vi "TX_ProdCons.vi"(8 "error in":errorcluster, 10 "queue in":refnum<queue>, 11 "Event Registration Refnum":refnum<event-registration>) -> (0 "error out":errorcluster)   [LabVIEW 2023]
uses:
  <vilib>/userDefined/High Color/IMAQdx.ctl
  TX_Control 3.ctl
  <vilib>/vision/Image Controls.llb/IMAQ Image.ctl
  TX_Cluster1TypeDef.ctl
  TX_EnumTypeDef.ctl
panel:
  in  "error in (no error)":errorcluster
  in  "Select Camera:":T1
  in  "EXIT":bool
  in  "Enable TCP":bool
  in  "Photo":bool
  in  "StartCam":bool
  in  "START":bool
  out "CamView":T2(plugin-control)
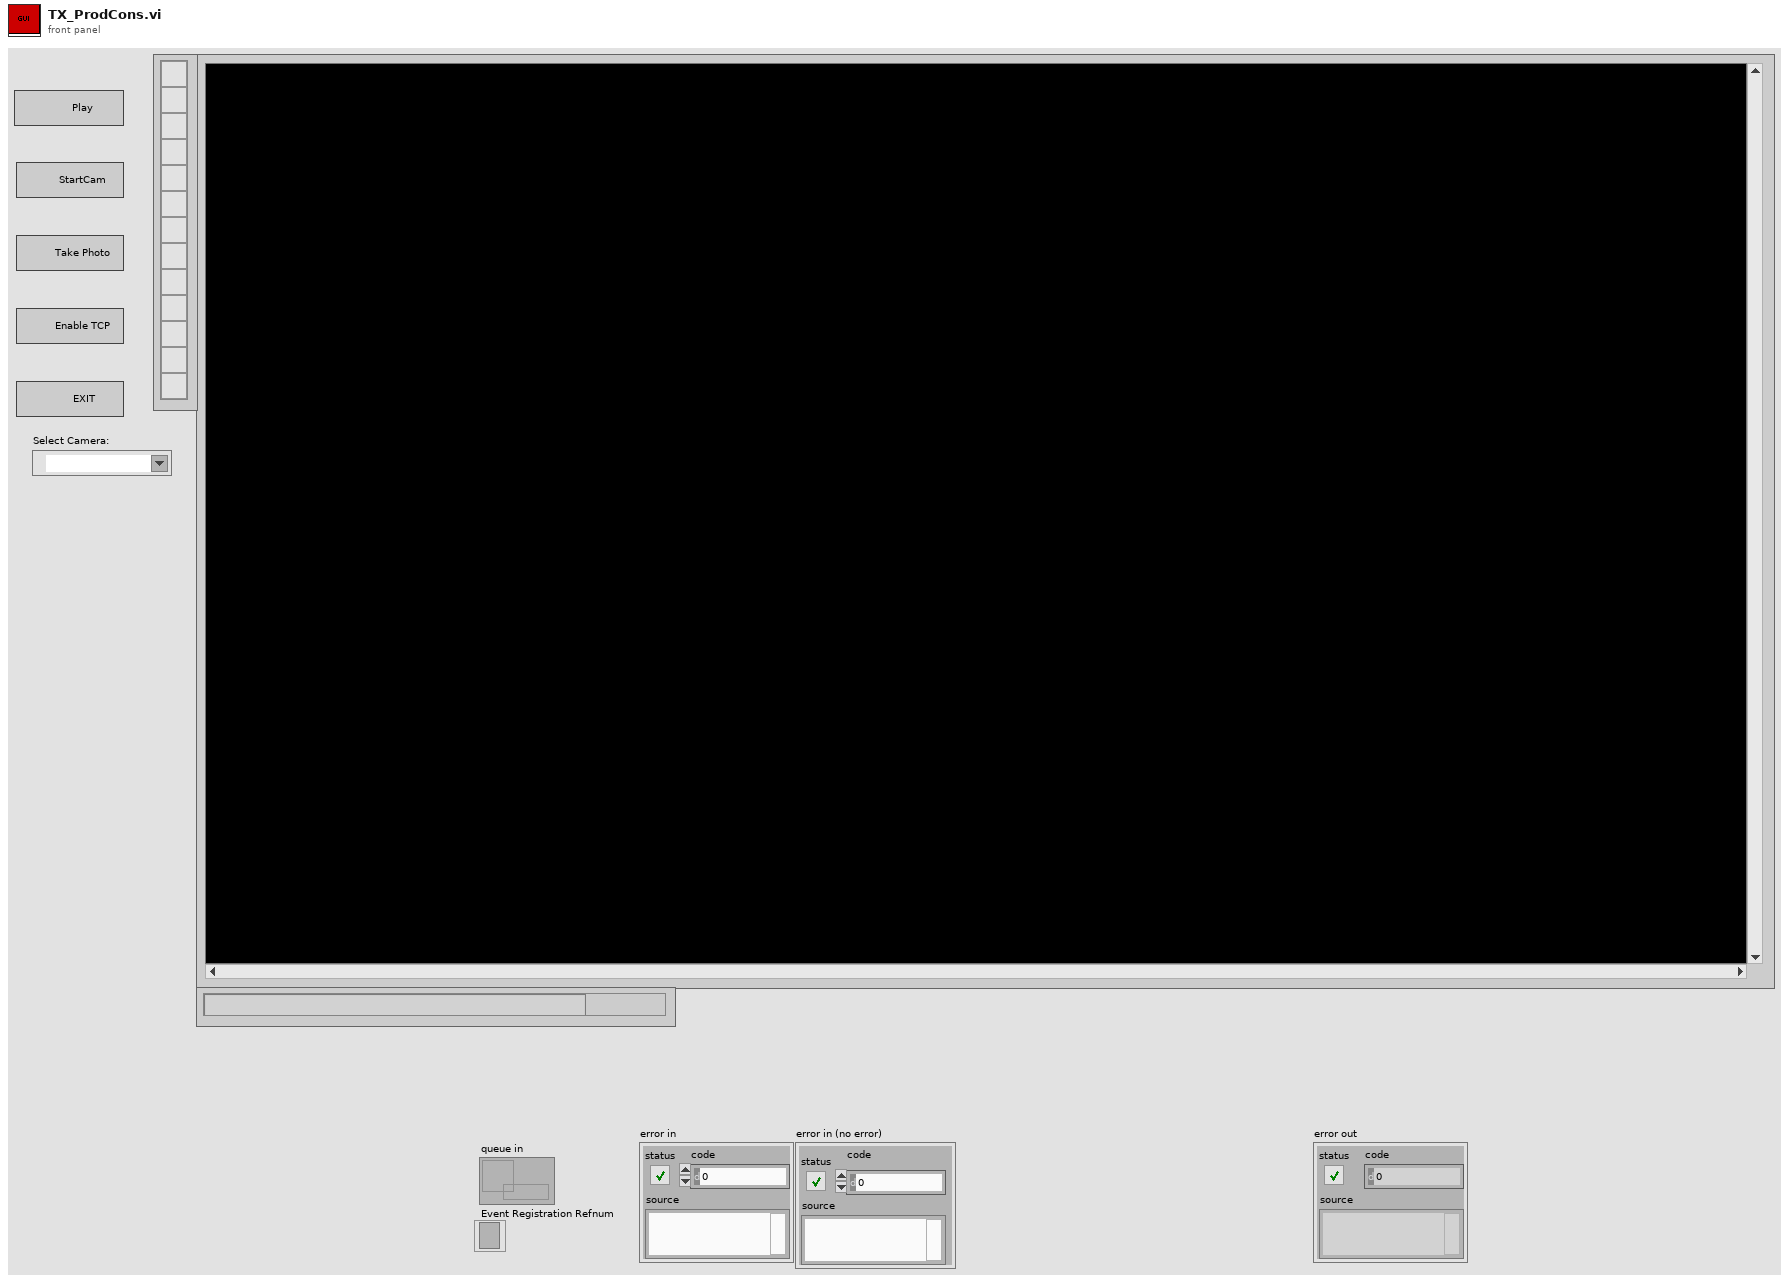
[diagram p1: front panel]
types:
  T1 = typedef "IMAQdx.ctl" = refnum<k21>
  T2 = typedef "IMAQ Image.ctl" = refnum<image>
  T3 = typedef "TX_EnumTypeDef.ctl" = enum16{"Initialize", "StartCam", "EnableTCP", "TakePhoto", "ShutDown"}
  T4 = cluster{"Enum":T3, "RawImage":T2, "Data":variant}
  T5 = typedef "TX_Cluster1TypeDef.ctl" = cluster{"Enum":T6, "CamSel":variant, "CamView":variant}
  T6 = typedef "TX_Control 3.ctl" = enum16{"Default", "StartCamera", "TakePhoto", "EnableTCP", "Cam2Display", "CloseAll"}
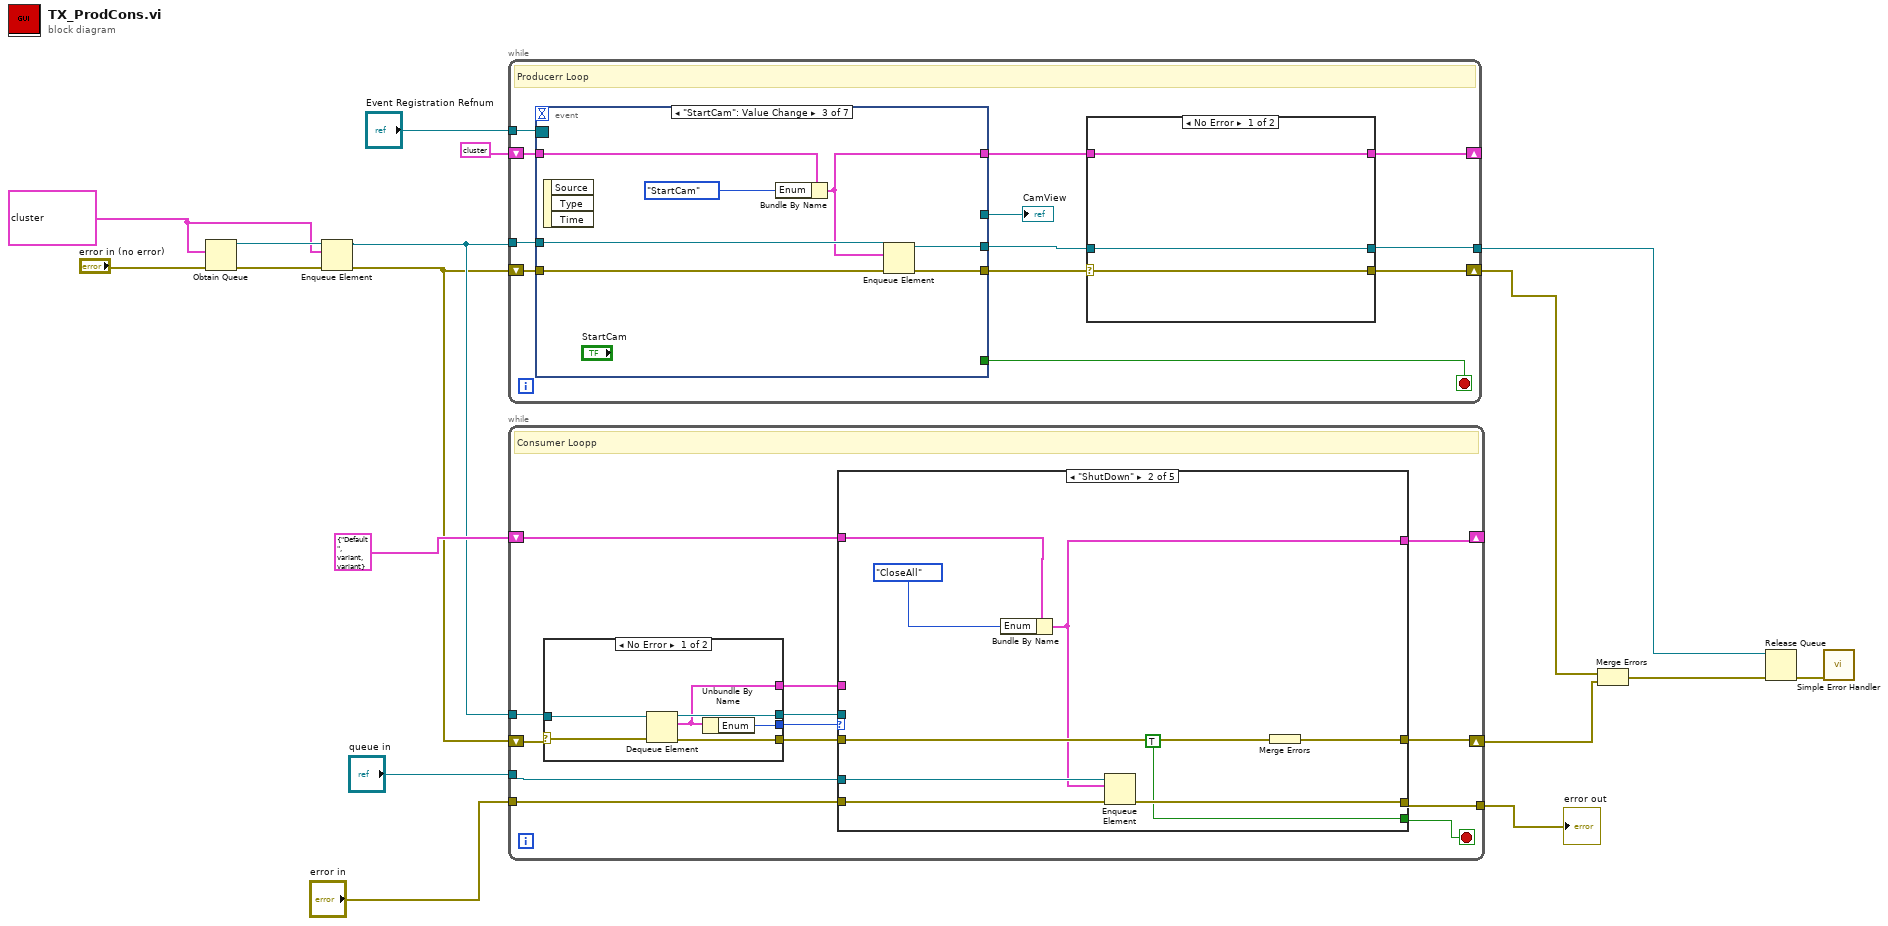
[diagram p0: block diagram]
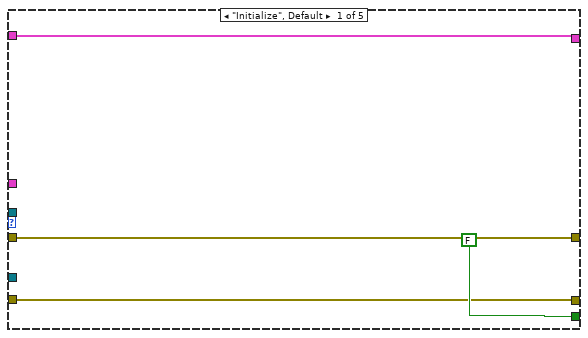
[diagram p2: hidden frame]
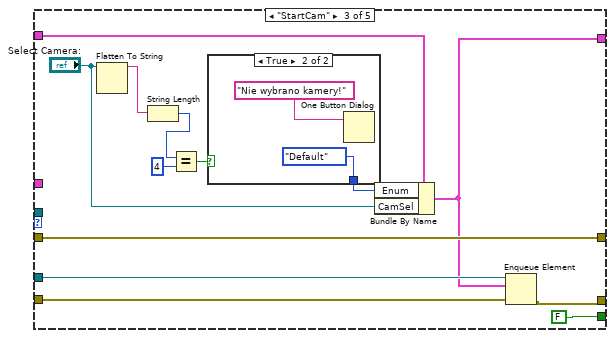
[diagram p3: hidden frame]
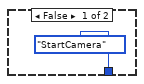
[diagram p4: hidden frame]
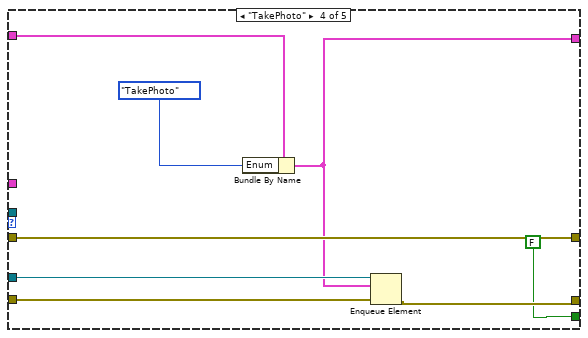
[diagram p5: hidden frame]
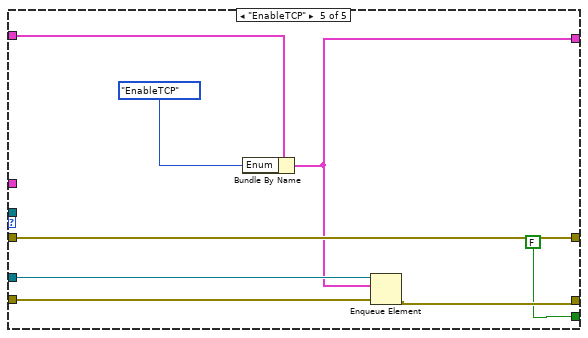
[diagram p6: hidden frame]
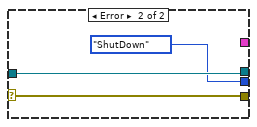
[diagram p7: hidden frame]
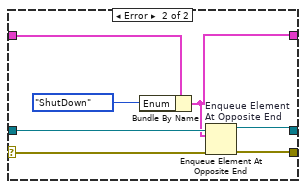
[diagram p8: hidden frame]
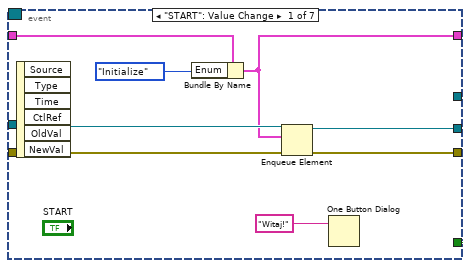
[diagram p9: hidden frame]
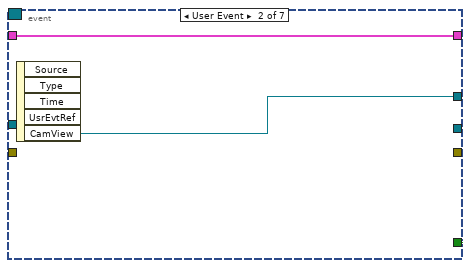
[diagram p10: hidden frame]
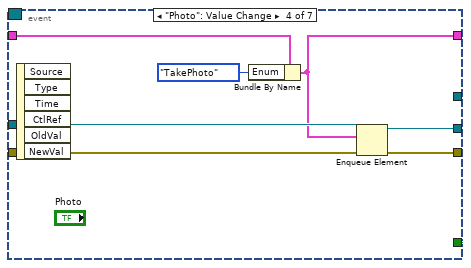
[diagram p11: hidden frame]
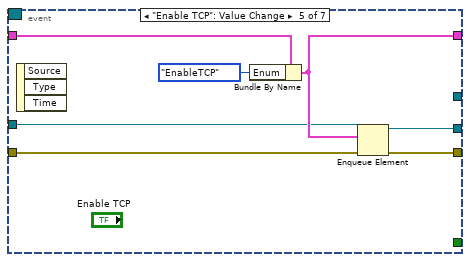
[diagram p12: hidden frame]
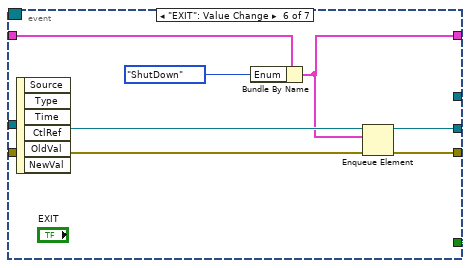
[diagram p13: hidden frame]
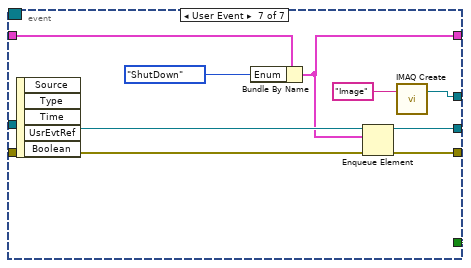
[diagram p14: hidden frame]
diagram:
  w10 = T4 {"Enum"=enum."Initialize", "RawImage"=refnum, "Data"=variant(refnum<image> refnum)} ("clusterSimple")
  n1 = Obtain Queue(element data type=w10, error in (no error)="error in (no error)") -> (queue out=w12:refnum<queue>, error out=w13:errorcluster)  [unwired: 3 in, 1 out]
  n2 = Enqueue Element(queue=w12, element=w10, error in (no error)=w13) -> (queue out=w9:refnum<queue>, error out=w8:errorcluster)  [unwired: 1 in, 1 out]
  n3 = while {
    shift-right: [w23] -> w5
    shift-left: w8 -> [w28]
    tunnel: w9 -> [w26]
    tunnel: [w24] -> w4
    tunnel: "Event Registration Refnum" -> [w22]
    shift-right: [w19] -> _
    shift-left: T4 {"Enum"=enum."Initialize", "RawImage"=refnum, "Data"=variant(refnum<image> refnum)} ("clusterSimple") -> [w21]
    stop <- w29 stop-if-true
    # "Producerr Loop"
    n4 = event shown="[2] \"StartCam\": Value Change" {
      selector: w22 -> [_ _ _ _ _ _ _]
      dyn-events: _ -> [_ _ _ _ _ _ _]
      timeout: _ -> [_ _ _ _ _ _ _]
      tunnel: [FALSE ("STOP") FALSE ("STOP") FALSE ("STOP") FALSE ("STOP") _ TRUE ("STOP") TRUE ("STOP")] -> w29
      tunnel: w28 -> [w47 _ w58 w66 w70 w82 w92]
      tunnel: [w46 _ w56 w64 w69 w81 w91] -> w27
      tunnel: w26 -> [w45 _ w59 w67 w71 w80 w90]
      tunnel: [w44 _ w57 w65 w68 w79 w89] -> w25
      tunnel: w21 -> [w43 w51 w55 w63 w72 w77 w87]
      tunnel: [w41 w51 w53 w62 w73 w75 w85] -> w20
      tunnel: [_ w49 _ _ _ _ w83] -> w18
      event "START": Value Change {
        n5 = event-data() -> ()  [unwired: 1 in, 6 out]
        n6 = Bundle By Name(cluster=w43, "Enum"=TX_EnumTypeDef."Initialize") -> (w41:T4)
        n7 = Enqueue Element(queue=w45, element=w41, error in (no error)=w47) -> (queue out=w44:refnum<queue>, error out=w46:errorcluster)  [unwired: 1 in, 1 out]
        n8 = One Button Dialog(message="Witaj!") -> ()  [unwired: 1 in, 1 out]
      }
      event User Event {
        n9 = event-data() -> ("CamView"=w49:T2)  [unwired: 1 in, 4 out]
      }
      event "StartCam": Value Change {
        n10 = event-data() -> ()  [unwired: 1 in, 3 out]
        n11 = Bundle By Name(cluster=w55, "Enum"=TX_EnumTypeDef."StartCam" ("element")) -> (w53:T4)
        n12 = Enqueue Element(queue=w59, element=w53, error in (no error)=w58) -> (queue out=w57:refnum<queue>, error out=w56:errorcluster)  [unwired: 1 in, 1 out]
      }
      event "Photo": Value Change {
        n13 = event-data() -> ()  [unwired: 1 in, 6 out]
        n14 = Bundle By Name(cluster=w63, "Enum"=TX_EnumTypeDef."TakePhoto") -> (w62:T4)
        n15 = Enqueue Element(queue=w67, element=w62, error in (no error)=w66) -> (queue out=w65:refnum<queue>, error out=w64:errorcluster)  [unwired: 1 in, 1 out]
      }
      event "Enable TCP": Value Change {
        n16 = event-data() -> ()  [unwired: 1 in, 3 out]
        n17 = Bundle By Name(cluster=w72, "Enum"=TX_EnumTypeDef."EnableTCP") -> (w73:T4)
        n18 = Enqueue Element(queue=w71, element=w73, error in (no error)=w70) -> (queue out=w68:refnum<queue>, error out=w69:errorcluster)  [unwired: 1 in, 1 out]
      }
      event "EXIT": Value Change {
        n19 = event-data() -> ()  [unwired: 1 in, 6 out]
        n20 = Bundle By Name(cluster=w77, "Enum"=TX_EnumTypeDef."ShutDown") -> (w75:T4)
        n21 = Enqueue Element(queue=w80, element=w75, error in (no error)=w82) -> (queue out=w79:refnum<queue>, error out=w81:errorcluster)  [unwired: 1 in, 1 out]
      }
      event User Event {
        n22 = event-data() -> ()  [unwired: 1 in, 5 out]
        n23 = Bundle By Name(cluster=w87, "Enum"=TX_EnumTypeDef."ShutDown") -> (w85:T4)
        n24 = Enqueue Element(queue=w90, element=w85, error in (no error)=w92) -> (queue out=w89:refnum<queue>, error out=w91:errorcluster)  [unwired: 1 in, 1 out]
        n25 = call "IMAQ Create"("Image Name"="Image") -> ("New Image"=w83:T2)  [unwired: 4 in, 1 out]
      }
    }
    "CamView" <- w18
    n26 = case shown="No Error" w27 {
      selector: w27 -> [w31 w39]
      tunnel: [w32 w36] -> w24
      tunnel: w25 -> [w32 w37]
      tunnel: [w31 w38] -> w23
      tunnel: w20 -> [w30 w34]
      tunnel: [w30 w33] -> w19
      frame No Error {
      }
      frame Error {
        n27 = Bundle By Name(cluster=w34, "Enum"=TX_EnumTypeDef."ShutDown") -> (w33:T4)
        n28 = Enqueue Element At Opposite End "Enqueue Element \nAt Opposite End"(queue=w37, element=w33, error in (no error)=w39) -> (queue out=w36:refnum<queue>, error out=w38:errorcluster)  [unwired: 1 in, 1 out]
      }
    }
  }
  n29 = while {
    shift-right: [w101] -> w3
    shift-left: w8 -> [w105]
    tunnel: w9 -> [w104]
    tunnel: "queue in" -> [w99]
    tunnel: "error in" -> [w98]
    tunnel: [w97] -> w17
    shift-right: [w95] -> _
    shift-left: T5 {"Enum"=enum."Default", "CamSel"=variant(refnum<image> refnum), "CamView"=variant(refnum<image> refnum)} ("Cluster") -> [w96]
    stop <- w93 stop-if-true
    # "Consumer Loopp"
    n30 = case shown="No Error" w105 {
      selector: w105 -> [w156 w159]
      tunnel: w104 -> [w154 w158]
      tunnel: [w155 w159] -> w102
      tunnel: [w153 w158] -> w100
      tunnel: [w152 TX_EnumTypeDef."ShutDown" ("Enum")] -> w103
      tunnel: [w151 _] -> w94
      frame No Error {
        n31 = Dequeue Element(queue=w154, error in (no error)=w156) -> (queue out=w153:refnum<queue>, element=w151:T4, error out=w155:errorcluster)  [unwired: 1 in, 1 out]
        n32 = Unbundle By Name(w151) -> ("Enum"=w152:T3)
      }
      frame Error {
      }
    }
    n33 = case shown="\"ShutDown\"" w103 {
      tunnel: w102 -> [w109 w118 w126 w137 w145]
      tunnel: [w109 w117 w126 w137 w145] -> w101
      tunnel: w100 -> [_ _ _ _ _]
      tunnel: [FALSE TRUE FALSE FALSE FALSE] -> w93
      tunnel: w99 -> [_ w112 w131 w142 w150]
      tunnel: w98 -> [w106 w114 w130 w141 w149]
      tunnel: [w106 w113 w129 w140 w148] -> w97
      tunnel: w96 -> [w107 w115 w127 w138 w146]
      tunnel: [w107 w110 w124 w135 w143] -> w95
      tunnel: w94 -> [_ _ _ _ _]
      frame "Initialize", Default {
      }
      frame "ShutDown" {
        n34 = Bundle By Name(cluster=w115, "Enum"=TX_Control_3."CloseAll") -> (w110:T5)
        n35 = Enqueue Element(queue=w112, element=w110, error in (no error)=w114) -> (error out=w113:errorcluster)  [unwired: 1 in, 2 out]
        n36 = Merge Errors(w118) -> (w117:errorcluster)
      }
      frame "StartCam" {
        n37 = Flatten To String(anything="Select Camera:") -> (data string=w122:string)  [unwired: 3 in, 2 out]
        n38 = String Length(string=w122) -> (length=w121:i32)
        n39 = Equal?(x=w121, y=4) -> (x = y?=w119:bool)
        n40 = case shown="True" w119 {
          tunnel: [TX_Control_3."StartCamera" ("Enum") TX_Control_3."Default" ("Enum")] -> w128
          frame False {
          }
          frame True {
            n41 = One Button Dialog(message="Nie wybrano kamery!") -> ()  [unwired: 1 in, 1 out]
          }
        }
        n42 = Bundle By Name(cluster=w127, "Enum"=w128, "CamSel"="Select Camera:") -> (w124:T5)
        n43 = Enqueue Element(queue=w131, element=w124, error in (no error)=w130) -> (error out=w129:errorcluster)  [unwired: 1 in, 2 out]
      }
      frame "TakePhoto" {
        n44 = Bundle By Name(cluster=w138, "Enum"=TX_Control_3."TakePhoto") -> (w135:T5)
        n45 = Enqueue Element(queue=w142, element=w135, error in (no error)=w141) -> (error out=w140:errorcluster)  [unwired: 1 in, 2 out]
      }
      frame "EnableTCP" {
        n46 = Bundle By Name(cluster=w146, "Enum"=TX_Control_3."EnableTCP") -> (w143:T5)
        n47 = Enqueue Element(queue=w150, element=w143, error in (no error)=w149) -> (error out=w148:errorcluster)  [unwired: 1 in, 2 out]
      }
    }
  }
  "error out" <- w17
  n48 = Merge Errors(w5, w3) -> (w7:errorcluster)
  n49 = Release Queue(queue=w4, error in (no error)=w7) -> (error out=w6:errorcluster)  [unwired: 1 in, 2 out]
  n50 = call <vilib>:"Simple Error Handler.vi"("error in (no error)"=w6) -> ()  [unwired: 4 in, 5 out]
